vi "Register-Based Template.vi"(8 "error in (no error)":errorcluster, 11 "VISA resource name":refnum<visa-resource-name>) -> (0 "error out":errorcluster, 3 "VISA resource name out":refnum<visa-resource-name>)   [LabVIEW 2011, in "Template - Register.lvlib"]
doc: "The Register-Based Template VI is used to create custom VIs. This VI includes basic elements of configuration and query VIs for register-based systems."
uses:
  <instrlib>/_Template - Register/Template - Register.lvlib
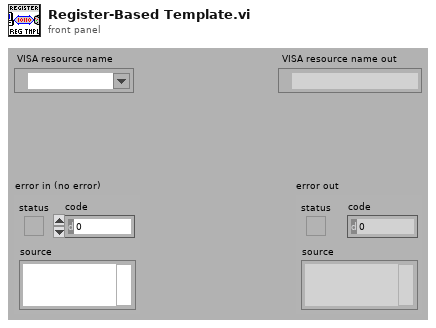
[diagram p1: front panel]
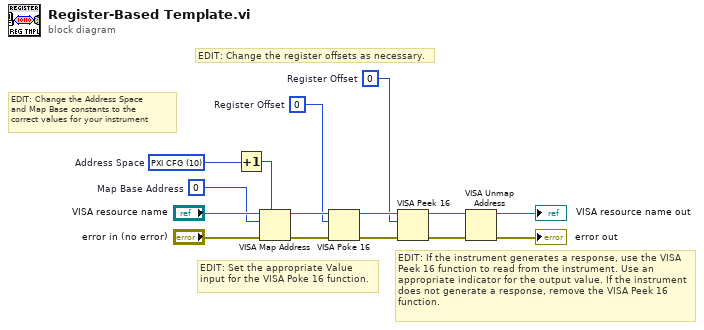
[diagram p0: block diagram]
diagram:
  w1 = u16 10 items=["A16"=1, "A24"=2, "A32"=3, "PXI CFG"=10, "PXI BAR0"=11, "PXI BAR1"=12, "PXI BAR2"=13, "PXI BAR3"=14, "PXI BAR4"=15, "PXI BAR5"=16]  # Address Space
  w4 = u32 0  # Register Offset
  w5 = u32 0  # Map Base Address
  w3 = u32 0  # Register Offset
  # "EDIT: Set the appropriate Value input for the VISA Poke 16 function."
  # "EDIT: If the instrument generates a response, use the VISA Peek 16 function to read from the instrument. Use an appropriate indicator for the output value. If the instrument does not generate a response, remove the VISA Peek 16 function."
  # "EDIT: Change the Address Space\nand Map Base constants to the\ncorrect values for your instrument"
  # "EDIT: Change the register offsets as necessary."
  n1 = Increment(x=w1) -> (x+1=w2:u16)
  n2 = VISA Map Address(7:w2, 8:"error in (no error)", 10:w5, 11:"VISA resource name") -> (0:w13:errorcluster, 3:w11:refnum<visa-resource-name>)  [unwired: 2 in]
  n3 = VISA Poke 16(8:w13, 10:w3, 11:w11) -> (0:w14:errorcluster, 3:w12:refnum<visa-resource-name>)  [unwired: 1 in]
  n4 = VISA Peek 16(8:w14, 10:w4, 11:w12) -> (0:w15:errorcluster, 3:w10:refnum<visa-resource-name>)  [unwired: 1 out]
  n5 = VISA Unmap Address(8:w15, 11:w10) -> (0:→"error out":errorcluster, 3:→"VISA resource name out":refnum<visa-resource-name>)
